vi "Load Effect.vi"(8 "error in (no error)":errorcluster, 9 "Effect Slot":i32, 10 "Effect Name":string, 11 "Effect Unit in":refnum<class "Effect Unit.lvclass">) -> (0 "error out":errorcluster, 3 "Effect Unit out":refnum<class "Effect Unit.lvclass">)   [LabVIEW 2019, in "Effect Unit.lvclass"]
uses:
  Effect Unit.lvclass
  Plugin Interfaces/Effect Interface/Effect Interface.lvlibp/Plugin Interfaces/Effect Interface/Effect Interface Class/Effect Interface.lvclass
  Effect Unit.lvclass/Effect Unit.ctl
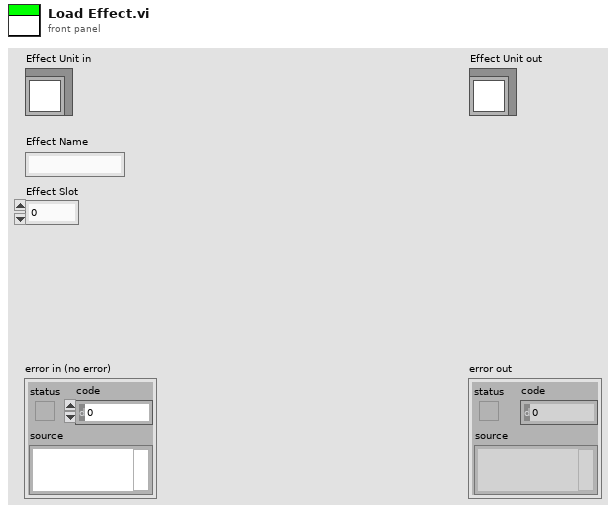
[diagram p1: front panel]
types:
  T1 = typedef "Effect Unit.lvclass/Effect Info.ctl" = cluster{"ID":string, "Message Queue":refnum<queue>, "Effect Interface":refnum<class "Effect Interface.lvclass">}
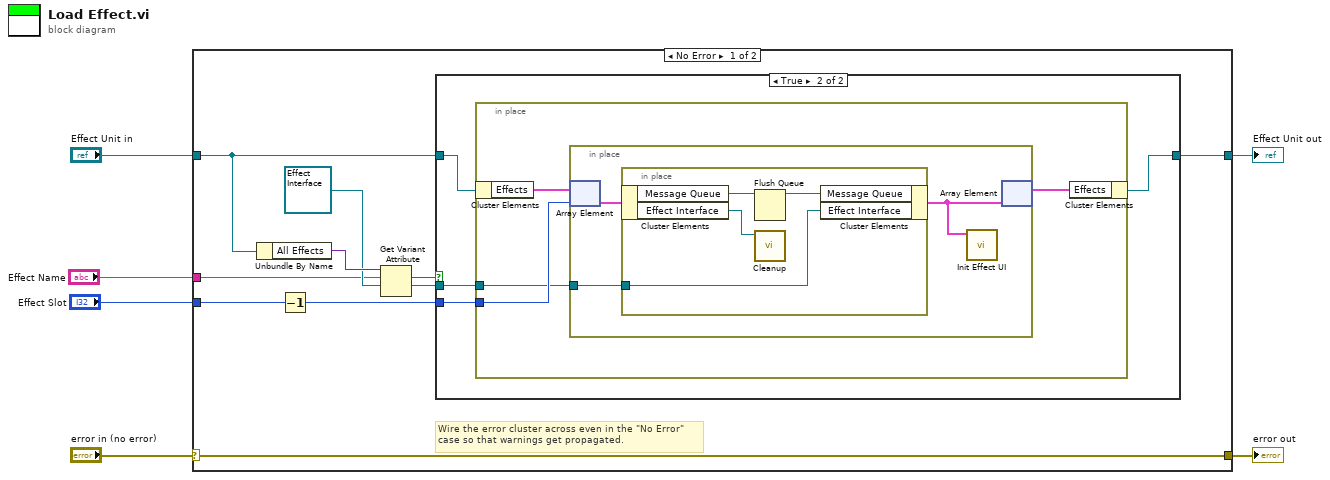
[diagram p0: block diagram]
diagram:
  n1 = case shown="No Error" "error in (no error)" {
    selector: "error in (no error)" -> [w16 w34]
    tunnel: [w16 w34] -> w5
    tunnel: [w9 w33] -> w3
    tunnel: "Effect Unit in" -> [w11 w33]
    tunnel: "Effect Name" -> [w7 _]
    tunnel: "Effect Slot" -> [w10 _]
    frame No Error {
      # "Wire the error cluster across even in the \"No Error\"\ncase so that warnings get propagated."
      n2 = Unbundle By Name(w11) -> ("All Effects"=w15:variant)
      n3 = Decrement(x=w10) -> (x-1=w8:i32)
      n4 = Get Variant Attribute(Variant=w15, name=w7, default value (empty Variant)=refnum<class "Effect Interface.lvclass"> refnum ("Effect Interface.lvlibp:Effect Interface.lvclass")) -> (found=w13:bool, value=w12:refnum<class "Effect Interface.lvclass">)  [unwired: 1 in, 2 out]
      n5 = case shown="True" w13 {
        tunnel: w12 -> [_ w19]
        tunnel: w11 -> [w17 w21]
        tunnel: w8 -> [_ w20]
        tunnel: [w17 w18] -> w9
        frame False {
        }
        frame True {
          n6 = in-place {
            in-place-border: w20 -> [w24]
            in-place-border: w19 -> [w23]
            n7 = in-place-cluster #1(w21) -> ("Effects"=w25:T1[])
            n8 = in-place {
              in-place-border: w23 -> [w27]
              n9 = in-place-array #2(w25, w24) -> (w28:T1)
              n10 = in-place {
                in-place-border: w27 -> [w31]
                n11 = in-place-cluster #3(w28) -> ("Message Queue"=w30:refnum<queue>, "Effect Interface"=w32:refnum<class "Effect Interface.lvclass">)
                n12 = Flush Queue(queue=w30) -> (queue out=w29:refnum<queue>)  [unwired: 1 in, 2 out]
                n13 = call-dynamic "Cleanup.vi"("Effect Interface in"=w32) -> ()  [unwired: 9 in, 2 out]
                n14 = in-place-cluster #3("Message Queue"=w29, "Effect Interface"=w31) -> (w26:T1)
              }
              n15 = call "Init Effect UI.vi"("Effect Info"=w26) -> ()  [unwired: 11 in]
              n16 = in-place-array #2(w26) -> (w22:T1[])  [unwired: 1 out]
            }
            n17 = in-place-cluster #1("Effects"=w22) -> (w18:refnum<class "Effect Unit.lvclass">)
          }
        }
      }
    }
    frame Error {
    }
  }
  "error out" <- w5
  "Effect Unit out" <- w3
